vi "Identities.vi"(8 "error in (no error)":errorcluster, 11 "TelemetryAPI in":refnum<class "TelemetryAPI.lvclass">) -> (0 "error out":errorcluster, 2 "Identities":refnum<class "Identity.lvclass">[](array[class]), 3 "TelemetryAPI out":refnum<class "TelemetryAPI.lvclass">)   [LabVIEW 2020, in "Volatus.lvlib" / "TelemetryAPI.lvclass"]
uses:
  TelemetryAPI.lvclass
  Identity/Identity.lvclass
  ApiIdentity/ApiIdentity.lvclass/ApiIdentity.ctl
  ApiIdentity/ApiIdentity.lvclass
  C:/dev/lv20CE/relink/lv-volatus/Volatus/Identity/Identity.lvclass
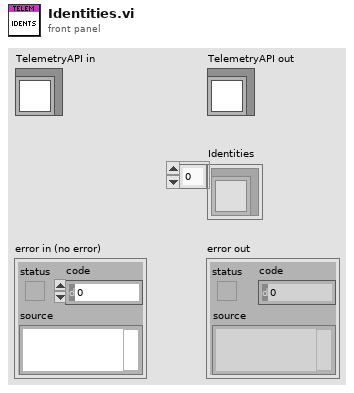
[diagram p1: front panel]
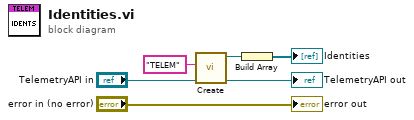
[diagram p0: block diagram]
diagram:
  n1 = call "Create.vi"("API ID"="TELEM") -> ("ApiIdentity out"=w3:refnum<class "ApiIdentity.lvclass">)  [unwired: 10 in]
  n2 = Build Array(w3) -> (→"Identities":refnum<class "ApiIdentity.lvclass">[])
  "error out" <- "error in (no error)"
  "TelemetryAPI out" <- "TelemetryAPI in"
